vi "image detect.vi"() -> ()   [LabVIEW 2012]
panel:
  in  "Burn Loops":i32
  out "Axis 2 (y axis)":dbl format="%.6f"
  out "Axis 1 x axis":dbl format="%.6f"
  in  "Relative Step Size":dbl
  in  "Axis in":i32=1
  out "Intensity Graph":dbl[][](graph)
  in  "Z Position":dbl
  in  "Coll. Time (sec)":dbl=4.0
  in  "No. Loops":i32
  in  "Save File path":path
  in  "Y Parameters":T1={"Number of Y Steps"=200, "Max Y (V)"=2.0, "Min Y (V)"=-2.0}
  in  "X Parameters":T2={"Number of X Steps"=200, "Max X (V)"=2.0, "Min X (V)"=-2.0}
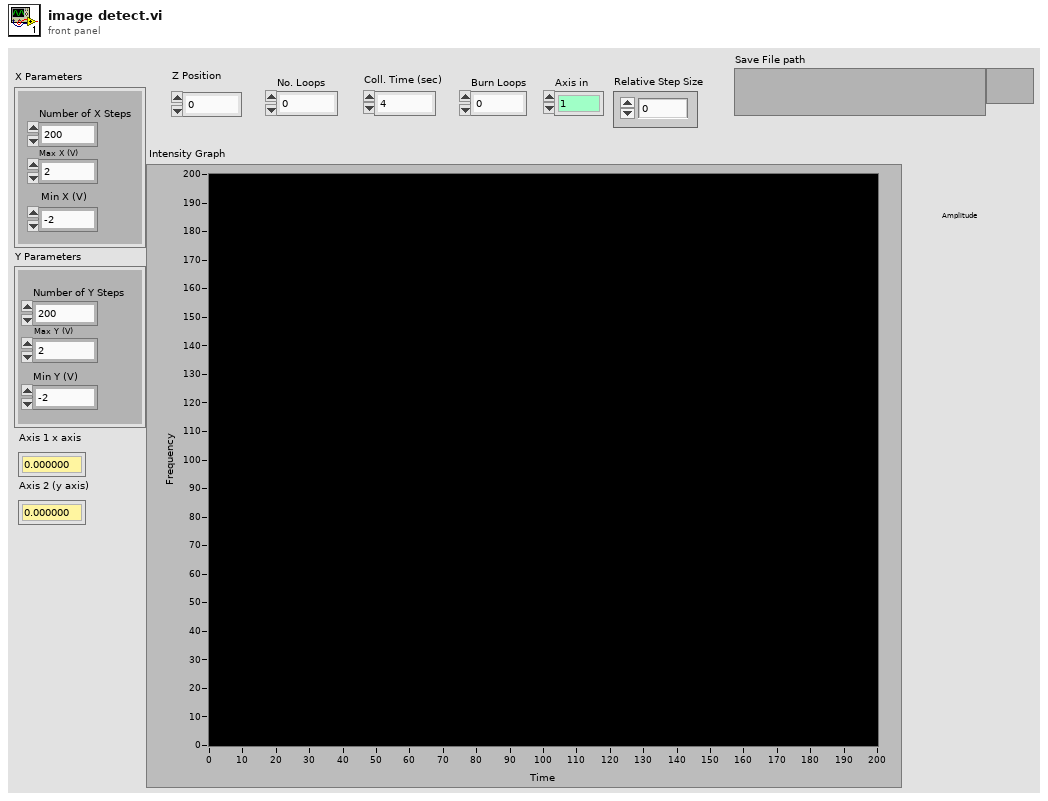
[diagram p1: front panel]
types:
  T1 = cluster{"Number of Y Steps":i32, "Max Y (V)":dbl, "Min Y (V)":dbl}
  T2 = cluster{"Number of X Steps":i32, "Max X (V)":dbl, "Min X (V)":dbl}
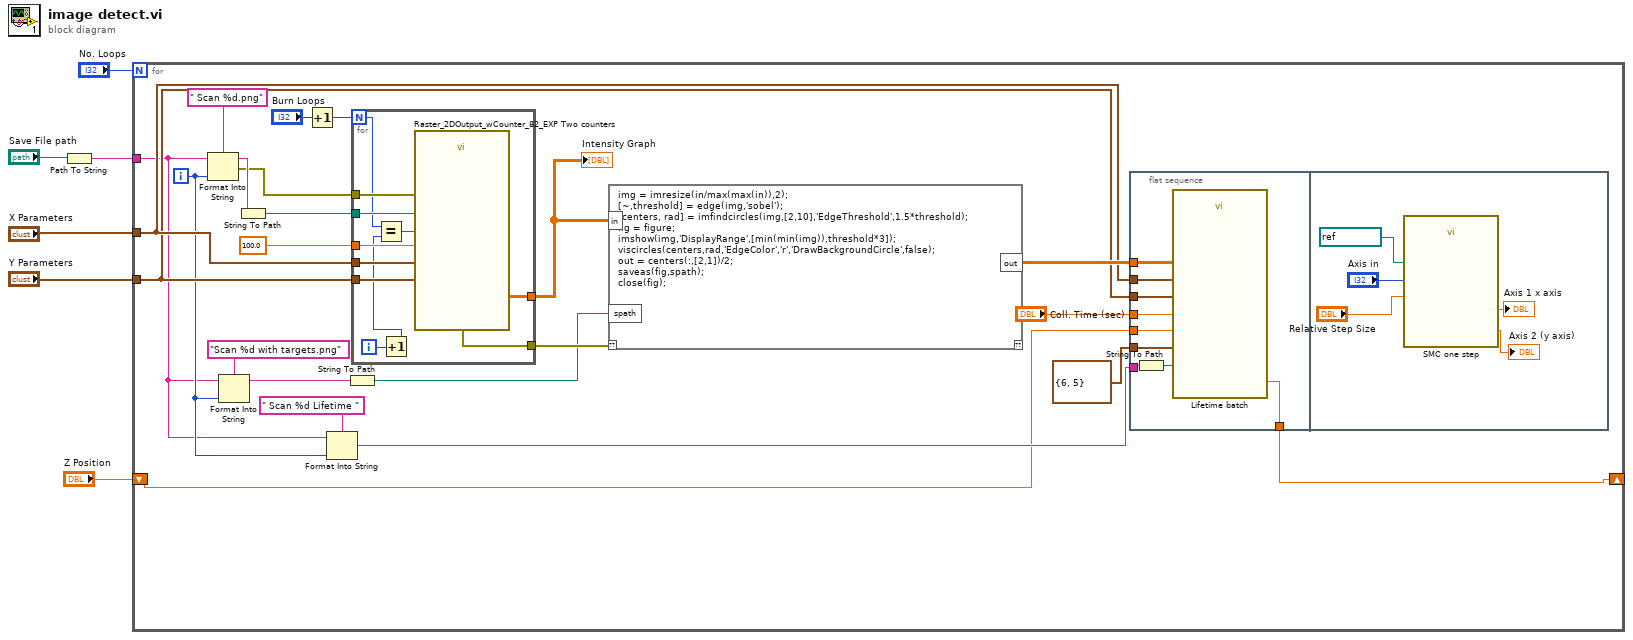
[diagram p0: block diagram]
diagram:
  n1 = Path To String(path="Save File path") -> (string=w2:string)
  n2 = for {
    N: "No. Loops" -> [_]
    tunnel: "X Parameters" -> [w19]
    tunnel: "Y Parameters" -> [w18]
    tunnel: w2 -> [w14]
    shift-right: [w9] -> _
    shift-left: "Z Position" -> [w10]
    i -> [w15]
    n3 = Format Into String(format string=" Scan %d.png", initial string=w14, w15) -> (resulting string=w25:string, error out=w24:errorcluster)  [unwired: 1 in]
    n4 = Format Into String(format string="Scan %d with targets.png", initial string=w14, w15) -> (resulting string=w22:string)  [unwired: 1 in, 1 out]
    n5 = String To Path(string=w25) -> (path=w26:path)
    n6 = Increment(x="Burn Loops") -> (x+1=w7:i32)
    n7 = Format Into String(format string=" Scan %d Lifetime ", initial string=w14, w15) -> (resulting string=w12:string)  [unwired: 1 in, 1 out]
    n8 = String To Path(string=w22) -> (path=w21:path)
    n9 = for {
      N: w7 -> [w30]
      tunnel: [w40] -> w29
      tunnel: 100.0 ("Update Rate (Hz)") -> [w39]
      tunnel: w26 -> [w38]
      tunnel: w24 -> [w37]
      tunnel: w19 -> [w36]
      tunnel: w18 -> [w35]
      tunnel: [w34] -> w11
      i -> [w32]
      n10 = Increment(x=w32) -> (x+1=w31:i32)
      n11 = Equal?(x=w30, y=w31) -> (x = y?=w33:bool)
      n12 = call "Raster_2DOutput_wCounter_82_EXP Two counters.vi"("Save File path"=w38, "Save?"=w33, "error in"=w37, "Update Rate (Hz)"=w39, "Y Parameters"=w35, "X Parameters"=w36) -> ("error out"=w40:errorcluster, "Intensity Graph"=w34:dbl[][])  [unwired: 2 in]
    }
    "Intensity Graph" <- w11
    n13 = script code="img = imresize(in/max(max(in)),2);\n[~,threshold] = edge(img,'sobel');\n[centers, rad] = imfindcircles(img,[2,10],'EdgeThreshold',1.5*threshold);\nfig = figure;\nimshow(img,'DisplayRange',[min(min(img)),threshold*3]);\nviscircles(centers,rad,'EdgeColor','r','DrawBackgroundCircle',false);\nout = centers(:,[2,1])/2;\nsaveas(fig,spath);\nclose(fig);"("??"=w29, "in"=w11, "spath"=w21) -> ("out"=w20:dbl[][])  [unwired: 1 out]
    n14 = flat-sequence {
      tunnel: w20 -> [w49]
      tunnel: w19 -> [w48]
      tunnel: w18 -> [w47]
      tunnel: "Coll. Time (sec)" -> [w46]
      tunnel: cluster{"Portnumber":i32, "Baudrate":u16} {"Portnumber"=6, "Baudrate"=5} ("RS232 settings") -> [w45]
      tunnel: w12 -> [w43]
      tunnel: [w42] -> w9
      tunnel: w10 -> [w41]
      frame #0 {
        n15 = String To Path(string=w43) -> (path=w44:path)
        n16 = call "Lifetime batch.vi"("Collection Time (seconds)"=w46, "File Path Control"=w44, "Array - Numeric"=w49, "Z Position"=w41, "RS232 settings"=w45, "Y Parameters"=w47, "X Parameters"=w48) -> ("Z Position 2"=w42:dbl)  [unwired: 4 in]
      }
      frame #1 {
        n17 = call "SMC one step.vi"("Relative Step Size"="Relative Step Size", "Axis in"="Axis in", "VISA Handle in"=refnum<visa-resource-name> "COM8") -> ("Axis 2 (y axis)"=→"Axis 2 (y axis)":dbl, "Axis 1 x axis"=→"Axis 1 x axis":dbl)  [unwired: 6 in, 1 out]
      }
    }
  }
